vi "Measurement.vi"() -> ()   [LabVIEW 2013]
uses:
  <vilib>/Utility/error.llb/DialogType.ctl
  <vilib>/DAQmx/write.llb/DAQmx Write (Digital 1D U32 1Chan NSamp).vi
  <vilib>/DAQmx/read.llb/DAQmx Read (Analog 1D DBL 1Chan NSamp).vi
  <vilib>/DAQmx/read.llb/DAQmx Read (Digital Wfm 1Chan NSamp).vi
  <vilib>/DAQmx/create/channels.llb/DAQmx Create Channel (DI-Digital Input).vi
  <vilib>/DAQmx/configure/timing.llb/DAQmx Timing (Sample Clock).vi
  <vilib>/DAQmx/configure/trigger.llb/DAQmx Start Trigger (Digital Edge).vi
  <vilib>/DAQmx/create/channels.llb/DAQmx Create Channel (AI-Voltage-Basic).vi
  <vilib>/DAQmx/create/channels.llb/DAQmx Create Channel (DO-Digital Output).vi
  <vilib>/DAQmx/create/channels.llb/DAQmx Create Channel (CO-Pulse Generation-Frequency).vi
  <vilib>/DAQmx/configure/timing.llb/DAQmx Timing (Implicit).vi
  <vilib>/DAQmx/miscellaneous.llb/DAQmx Fill In Error Info.vi
  <vilib>/Waveform/DWDTOps.llb/DWDT Digital to Analog.vi
  <resource>/objmgr/daqmx.rc
panel:
  out "Stop":bool=TRUE
  in  "DigitalOutputChannel":tag="Dev1/port0/line0:1"
  out "DO.ActualFreq":dbl=6000.0 format="%#.4f"
  out "CO.Actual Duty Cycle":dbl=0.5
  out "CO.ActualFreq":dbl=6000.240009600384 format="%#.4f"
  in  "SampleClockRate":dbl=1000.0 format="%#.4f"
  in  "CounterOutputTerminal":tag="/Dev1/PFI12"
  in  "CounterDevice":tag="Dev1/ctr0"
  out "Waveform Graph":waveform(dbl)[](graph)=[{"t0"=timestamp(0 s since 1904-01-01), "dt"=0.0005, "Y"=array[2000 elements]}, {"t0"=timestamp(0 s since 1904-01-01), "dt"=0.0005, "Y"=array[2000 elements]}, {"t0"=timestamp(0 s since 1904-01-01), "dt"=0.0005, "Y"=array[2000 elements]}]
  in  "Sample Clock Source":tag="/Dev1/PFI0"
  in  "AIChannel":tag="Dev1/ai0"
  out "AI.ActualFreq":dbl=6000.0 format="%#.4f"
  in  "Stop":bool
  out "DI.ActualFreq":dbl=6000.0 format="%#.4f"
  in  "DigitalInputChannel":tag="Dev1/port0/line3:2"
  # "使用設備\nUSB-6351\n\nMEMS加速規型號\nKXPA4\n\n接線表\nKXPA4       6351\n----------------------\nVmux         AI 0\nVCC            5V \nPS               5V\nST               DGND / AGND\nGND          DGND / AGND\nS0               p0.0 / p0.2\nS1               p0.1 / p0.3"
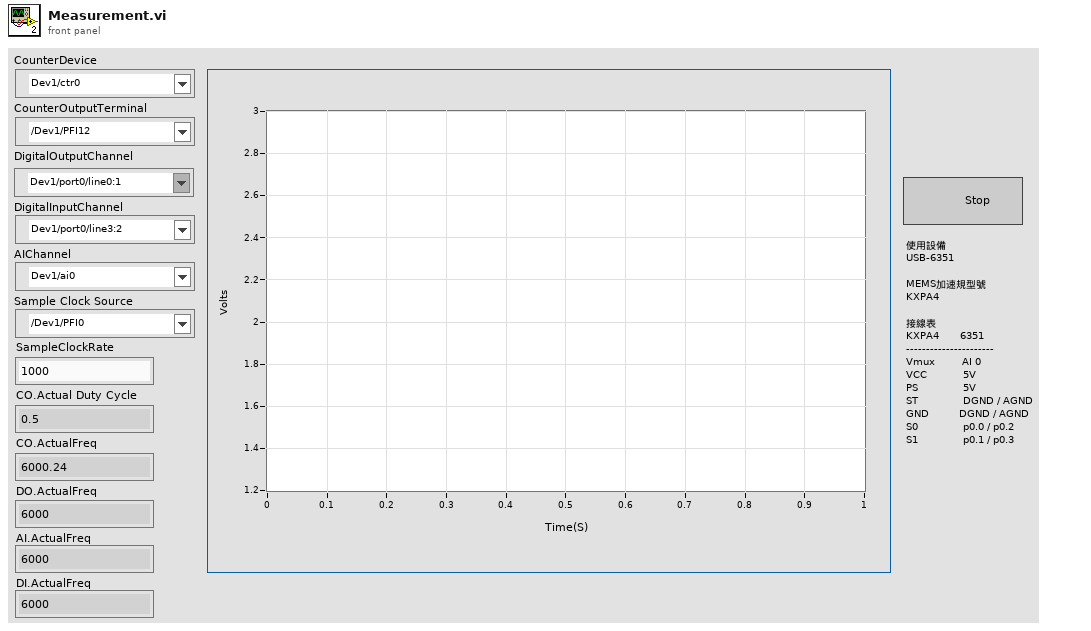
[diagram p1: front panel]
types:
  T1 = typedef "DialogType.ctl" = u16
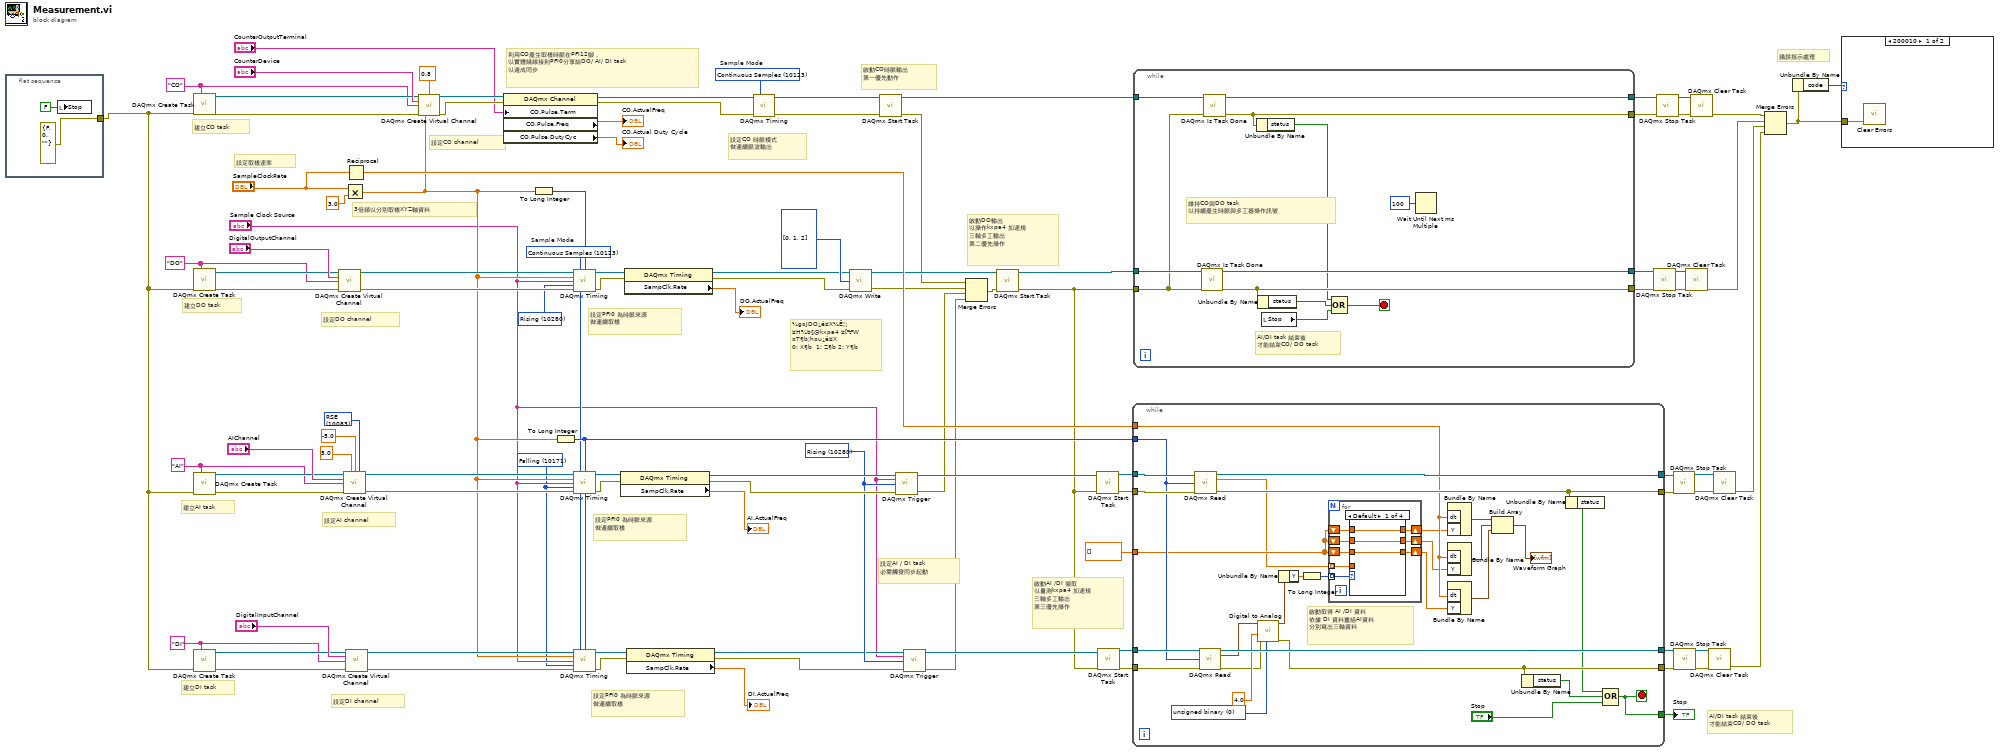
[diagram p0: block diagram]
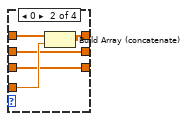
[diagram p2: hidden frame]
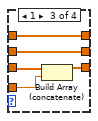
[diagram p3: hidden frame]
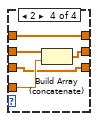
[diagram p4: hidden frame]
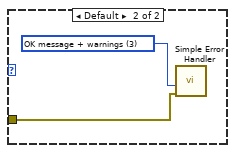
[diagram p5: hidden frame]
diagram:
  w1 = 10280 items=["Rising"=10280, "Falling"=10171] ("active edge")
  w2 = 10171 items=["Rising"=10280, "Falling"=10171] ("active edge")
  w6 = "DI" ("name to assign")
  w7 = "AI" ("name to assign")
  w5 = "CO" ("name to assign")
  w12 = "DO" ("name to assign")
  w81 = 10083 items=["default"=-1, "RSE"=10083, "NRSE"=10078, "Differential"=10106, "Pseudodifferential"=12529] ("Terminal Configuration")
  w66 = 10123 items=["Finite Samples"=10178, "Continuous Samples"=10123, "Hardware Timed Single Point"=12522]  # Sample Mode
  w72 = 10280 items=["Rising"=10280, "Falling"=10171] ("edge")
  w26 = 10123 items=["Finite Samples"=10178, "Continuous Samples"=10123, "Hardware Timed Single Point"=12522]  # Sample Mode
  # "錯誤指示處理"
  # "AI/DI task 結束後\n才能結束CO/ DO task"
  # "啟動AI /DI 擷取\n以量測kxpa4 加速規\n三軸多工輸出\n第三優先操作"
  # "啟動DO輸出\n以操作kxpa4 加速規\n三軸多工輸出\n第二優先操作"
  # "設定AI / DI task\n必需觸發同步起動"
  # "¼g¤JDO¿é¥X¼Ë¦¡\n¥H¾Þ§@kxpa4 ¥[³t³W\n¤T¶b¦h¤u¿é¥X\n0: X¶b  1: Z¶b 2: Y¶b"
  # "啟動CO時脈輸出\n第一優先動作"
  # "設定CO 時脈模式\n做連續脈波輸出"
  # "設定PFI0 為時脈來源\n做連續取樣"
  # "設定PFI0 為時脈來源\n做連續取樣"
  # "設定PFI0 為時脈來源\n做連續取樣"
  # "利用CO產生取樣時脈在PFI12腳，\n以實體繞線接到PFI0分享給DO/ AI/ DI task \n以達成同步"
  # "3倍頻以分別取樣XYZ軸資料"
  # "設定取樣速率"
  # "設定CO channel"
  # "設定DO channel"
  # "設定AI channel"
  # "設定DI channel"
  # "建立DI task"
  # "建立AI task"
  # "建立DO task"
  # "建立CO task"
  n1 = flat-sequence {
    tunnel: [errorcluster {"status"=FALSE, "code"=0, "source"=""} ("error in")] -> w3
    frame #0 {
      n2 = local write "Stop"(FALSE ("Stop")) -> ()
    }
  }
  n3 = call <vilib>:"DAQmx Create Task.vi"("new task name"=w5, "error in"=w3) -> ("task out"=w15:refnum<k21>, "error out"=w16:errorcluster)  [unwired: 12 in]
  n4 = call <vilib>:"DAQmx Create Task.vi"("new task name"=w12, "error in"=w3) -> ("task out"=w14:refnum<k21>, "error out"=w13:errorcluster)  [unwired: 12 in]
  n5 = call <vilib>:"DAQmx Create Task.vi"("new task name"=w7, "error in"=w3) -> ("task out"=w11:refnum<k21>, "error out"=w10:errorcluster)  [unwired: 12 in]
  n6 = call <vilib>:"DAQmx Create Task.vi"("new task name"=w6, "error in"=w3) -> ("task out"=w9:refnum<k21>, "error out"=w8:errorcluster)  [unwired: 12 in]
  n7 = call-poly <vilib>:"DAQmx Create Virtual Channel.vi"("task in"=w14, "lines"="DigitalOutputChannel", "name to assign"=w12, "error in"=w13) -> ("task out"=w50:refnum<k21>, "error out"=w49:errorcluster)  [unwired: 10 in]
  n8 = call-poly <vilib>:"DAQmx Create Virtual Channel.vi"("task in"=w11, "maximum value"=5.0 ("Max Voltage"), "minimum value"=-5.0 ("Min Voltage"), "input terminal configuration"=w81, "physical channels"="AIChannel", "name to assign"=w7, "error in"=w10) -> ("task out"=w87:refnum<k21>, "error out"=w88:errorcluster)  [unwired: 7 in]
  n9 = Multiply(x="SampleClockRate", y=3.0) -> (x*y=w24:dbl)
  n10 = Reciprocal(x="SampleClockRate") -> (1/x=w67:dbl)
  n11 = call-poly <vilib>:"DAQmx Create Virtual Channel.vi"("task in"=w9, "lines"="DigitalInputChannel", "name to assign"=w6, "error in"=w8) -> ("task out"=w102:refnum<k21>, "error out"=w101:errorcluster)  [unwired: 10 in]
  n12 = call-poly <vilib>:"DAQmx Create Virtual Channel.vi"("task in"=w15, "frequency"=w24, "duty cycle"=0.8, "counter"="CounterDevice", "name to assign"=w5, "error in"=w16) -> ("task out"=w63:refnum<k21>, "error out"=w62:errorcluster)  [unwired: 8 in]
  n13 = property class="DAQmx Channel"(reference=w63, error in=w62, "CO.Pulse.Term"="CounterOutputTerminal") -> (reference out=w59:refnum<k21>, error out=w60:errorcluster, "CO.Pulse.Freq"=→"CO.ActualFreq":dbl, "CO.Pulse.DutyCyc"=→"CO.Actual Duty Cycle":dbl)
  n14 = To Long Integer(number=w24) -> (32bit integer=w35:i32)
  n15 = To Long Integer(number=w24) -> (32bit integer=w69:i32)
  n16 = call-poly <vilib>:"DAQmx Timing.vi"("task/channels in"=w50, "sample mode"=w26, "samples per channel"=w35, "rate"=w24, "source"="Sample Clock Source", "active edge"=w1, "error in"=w49) -> ("task out"=w48:refnum<k21>, "error out"=w47:errorcluster)  [unwired: 7 in]
  n17 = call-poly <vilib>:"DAQmx Timing.vi"("task/channels in"=w87, "sample mode"=w26, "samples per channel"=w69, "rate"=w24, "source"="Sample Clock Source", "active edge"=w2, "error in"=w88) -> ("task out"=w90:refnum<k21>, "error out"=w89:errorcluster)  [unwired: 7 in]
  n18 = call-poly <vilib>:"DAQmx Timing.vi"("task/channels in"=w102, "sample mode"=w26, "samples per channel"=w69, "rate"=w24, "source"="Sample Clock Source", "active edge"=w2, "error in"=w101) -> ("task out"=w100:refnum<k21>, "error out"=w99:errorcluster)  [unwired: 7 in]
  n19 = property class="DAQmx Timing"(reference=w90, error in=w89) -> (reference out=w74:refnum<k21>, error out=w73:errorcluster, "SampClk.Rate"=→"AI.ActualFreq":dbl)
  n20 = property class="DAQmx Timing"(reference=w48, error in=w47) -> (reference out=w37:refnum<k21>, error out=w36:errorcluster, "SampClk.Rate"=→"DO.ActualFreq":dbl)
  n21 = property class="DAQmx Timing"(reference=w100, error in=w99) -> (reference out=w71:refnum<k21>, error out=w70:errorcluster, "SampClk.Rate"=→"DI.ActualFreq":dbl)
  n22 = call-poly <vilib>:"DAQmx Timing.vi"("task/channels in"=w59, "sample mode"=w66, "error in"=w60) -> ("task out"=w52:refnum<k21>, "error out"=w51:errorcluster)  [unwired: 11 in]
  n23 = call-poly <vilib>:"DAQmx Write.vi"("task/channels in"=w37, "data"=u32[] [0, 1, 2] ("Output Array"), "error in"=w36) -> ("task out"=w44:refnum<k21>, "error out"=w34:errorcluster)  [unwired: 10 in, 1 out]
  n24 = call <vilib>:"DAQmx Start Task.vi"("task/channels in"=w52, "error in"=w51) -> ("task out"=w65:refnum<k21>, "error out"=w33:errorcluster)  [unwired: 12 in]
  n25 = call-poly <vilib>:"DAQmx Trigger.vi"("task/channels in"=w74, "source"="Sample Clock Source", "edge"=w72, "error in"=w73) -> ("task out"=w86:refnum<k21>, "error out"=w21:errorcluster)  [unwired: 10 in]
  n26 = call-poly <vilib>:"DAQmx Trigger.vi"("task/channels in"=w71, "source"="Sample Clock Source", "edge"=w72, "error in"=w70) -> ("task out"=w97:refnum<k21>, "error out"=w20:errorcluster)  [unwired: 10 in]
  n27 = Merge Errors(w33, w34, w21, w20) -> (w32:errorcluster)
  n28 = call <vilib>:"DAQmx Start Task.vi"("task/channels in"=w44, "error in"=w32) -> ("task out"=w43:refnum<k21>, "error out"=w19:errorcluster)  [unwired: 12 in]
  n29 = call <vilib>:"DAQmx Start Task.vi"("task/channels in"=w86, "error in"=w19) -> ("task out"=w85:refnum<k21>, "error out"=w84:errorcluster)  [unwired: 12 in]
  n30 = call <vilib>:"DAQmx Start Task.vi"("task/channels in"=w97, "error in"=w19) -> ("task out"=w95:refnum<k21>, "error out"=w96:errorcluster)  [unwired: 12 in]
  n31 = while {
    tunnel: w96 -> [w135]
    tunnel: w95 -> [w134]
    tunnel: [w133] -> w92
    tunnel: [w132] -> w91
    tunnel: w85 -> [w131]
    tunnel: w84 -> [w130]
    tunnel: [w129] -> w78
    tunnel: [w128] -> w77
    tunnel: w69 -> [w127]
    tunnel: dbl[] [] ("data") -> [w126]
    tunnel: w67 -> [w125]
    tunnel: [w106] -> w4
    stop <- w106 stop-if-true
    w124 = u16 0 items=["unsigned binary", "offset binary", "2's complement"] ("data format (offset binary)")
    # "啟動取得 AI /DI 資料\n依據 DI 資料重組AI資料\n分別寫出三軸資料"
    n32 = call-poly <vilib>:"DAQmx Read.vi"("task/channels in"=w131, "number of samples per channel"=w127, "error in"=w130) -> ("task out"=w129:refnum<k21>, "data"=w117:dbl[], "error out"=w128:errorcluster)  [unwired: 10 in]
    n33 = call-poly <vilib>:"DAQmx Read.vi"("task/channels in"=w134, "number of samples per channel"=w127, "error in"=w135) -> ("task out"=w133:refnum<k21>, "data"=w123:digitalwaveform, "error out"=w121:errorcluster)  [unwired: 10 in]
    n34 = call-poly <vilib>:"Digital to Analog.vi"("data format (offset binary)"=w124, "error in (no error)"=w121, "full-scale range (pk-pk)"=4.0, "digital waveform"=w123) -> ("error out"=w132:errorcluster, "analog waveform"=w120:waveform(dbl))  [unwired: 4 in, 2 out]
    n35 = Unbundle By Name(w120) -> ("Y"=w119:dbl[])
    n36 = To Long Integer(number=w119) -> (32bit integer=w118:i32[])
    n37 = for {
      tunnel: w118 -> [w143] mode=indexing
      tunnel: w117 -> [w142] mode=indexing
      shift-right: [w140] -> w116
      shift-left: w126 -> [w141]
      shift-right: [w139] -> w115
      shift-left: w126 -> [w138]
      shift-right: [w137] -> w114
      shift-left: w126 -> [w136]
      n38 = case shown="Default" w143 {
        tunnel: w142 -> [_ w149 w153 w160]
        tunnel: w141 -> [w146 w151 w156 w161]
        tunnel: [w146 w150 w156 w161] -> w140
        tunnel: [w145 w148 w152 w158] -> w139
        tunnel: w138 -> [w145 w148 w152 w159]
        tunnel: [w144 w147 w154 w157] -> w137
        tunnel: w136 -> [w144 w147 w155 w157]
        frame Default {
        }
        frame 0 {
          n39 = Build Array (concatenate)(w151, w149) -> (w150:dbl[])
        }
        frame 1 {
          n40 = Build Array (concatenate)(w155, w153) -> (w154:dbl[])
        }
        frame 2 {
          n41 = Build Array (concatenate)(w159, w160) -> (w158:dbl[])
        }
      }
    }
    n42 = Bundle By Name("dt"=w125, "Y"=w116) -> (w113:waveform(dbl))  [unwired: 1 in]
    n43 = Bundle By Name("dt"=w125, "Y"=w115) -> (w112:waveform(dbl))  [unwired: 1 in]
    n44 = Bundle By Name("dt"=w125, "Y"=w114) -> (w111:waveform(dbl))  [unwired: 1 in]
    n45 = Build Array(w113, w112, w111) -> (→"Waveform Graph":waveform(dbl)[])
    n46 = Unbundle By Name(w132) -> ("status"=w108:bool)
    n47 = Unbundle By Name(w128) -> ("status"=w109:bool)
    n48 = Compound Arithmetic op=OR(w109, w108, "Stop") -> (w106:bool)
  }
  "Stop" <- w4
  n49 = while {
    tunnel: w65 -> [w173]
    tunnel: [w172] -> w54
    tunnel: [w171] -> w53
    tunnel: w43 -> [w170]
    tunnel: [w169] -> w39
    tunnel: [w168] -> w38
    tunnel: w19 -> [w167]
    stop <- w162 stop-if-true
    # "AI/DI task 結束後\n才能結束CO/ DO task"
    # "維持CO與DO task \n以持續產生時脈與多工器操作訊號"
    n50 = call <vilib>:"DAQmx Is Task Done.vi"("task/channels in"=w170, "error in"=w167) -> ("task out"=w169:refnum<k21>, "error out"=w168:errorcluster)  [unwired: 11 in, 1 out]
    n51 = call <vilib>:"DAQmx Is Task Done.vi"("task/channels in"=w173, "error in"=w167) -> ("task out"=w172:refnum<k21>, "error out"=w171:errorcluster)  [unwired: 11 in, 1 out]
    n52 = Unbundle By Name(w171) -> ("status"=w166:bool)
    n53 = Unbundle By Name(w168) -> ("status"=w165:bool)
    n54 = local read "Stop"() -> (w164:bool)
    n55 = Compound Arithmetic op=OR(w166, w165, w164) -> (w162:bool)
    n56 = Wait Until Next ms Multiple(millisecond multiple=u32 100) -> ()  [unwired: 1 out]
  }
  n57 = call <vilib>:"DAQmx Stop Task.vi"("task/channels in"=w39, "error in"=w38) -> ("task out"=w41:refnum<k21>, "error out"=w40:errorcluster)  [unwired: 12 in]
  n58 = call <vilib>:"DAQmx Stop Task.vi"("task/channels in"=w54, "error in"=w53) -> ("task out"=w56:refnum<k21>, "error out"=w55:errorcluster)  [unwired: 12 in]
  n59 = call <vilib>:"DAQmx Stop Task.vi"("task/channels in"=w78, "error in"=w77) -> ("task out"=w75:refnum<k21>, "error out"=w76:errorcluster)  [unwired: 12 in]
  n60 = call <vilib>:"DAQmx Stop Task.vi"("task/channels in"=w92, "error in"=w91) -> ("task out"=w94:refnum<k21>, "error out"=w93:errorcluster)  [unwired: 12 in]
  n61 = call <vilib>:"DAQmx Clear Task.vi"("task in"=w41, "error in"=w40) -> ("error out"=w31:errorcluster)  [unwired: 13 in]
  n62 = call <vilib>:"DAQmx Clear Task.vi"("task in"=w56, "error in"=w55) -> ("error out"=w30:errorcluster)  [unwired: 13 in]
  n63 = call <vilib>:"DAQmx Clear Task.vi"("task in"=w94, "error in"=w93) -> ("error out"=w17:errorcluster)  [unwired: 13 in]
  n64 = call <vilib>:"DAQmx Clear Task.vi"("task in"=w75, "error in"=w76) -> ("error out"=w18:errorcluster)  [unwired: 13 in]
  n65 = Merge Errors(w30, w31, w18, w17) -> (w29:errorcluster)
  n66 = Unbundle By Name(w29) -> ("code"=w28:i32)
  n67 = case shown="200010" w28 {
    tunnel: w29 -> [w174 w175]
    frame 200010 {
      n68 = call <vilib>:"Clear Errors.vi"("error in (no error)"=w174) -> ()  [unwired: 6 in, 1 out]
    }
    frame Default {
      w176 = T1 3 items=["no dialog", "OK message", "continue or stop message", "OK message + warnings", "continue/stop + warnings"] ("type of dialog (OK msg:1)")
      n69 = call <vilib>:"Simple Error Handler.vi"("type of dialog (OK msg:1)"=w176, "error in (no error)"=w175) -> ()  [unwired: 3 in, 5 out]
    }
  }
